vi "Housekeeping of Plugins.vi"(8 "error in (no error)":errorcluster, 11 "CIFPluginManager in":refnum<class "CIFPluginManager.lvclass">) -> (0 "error out":errorcluster)   [LabVIEW 2021, in "CIFPluginManager.lvclass"]
uses:
  CIFPluginManager.lvclass
  CIFPluginManager.lvclass/CIFPluginManager.ctl
  <vilib>/Utility/miscctls.llb/LVMapReplaceAction.ctl
  <vilib>/CIF Foundation/CIF Utilities/Time/System Time/LabVIEW Time to TAI Time.vi
  <vilib>/CIF Foundation/CIF Utilities/Time/Time_CIF_U.lvlib
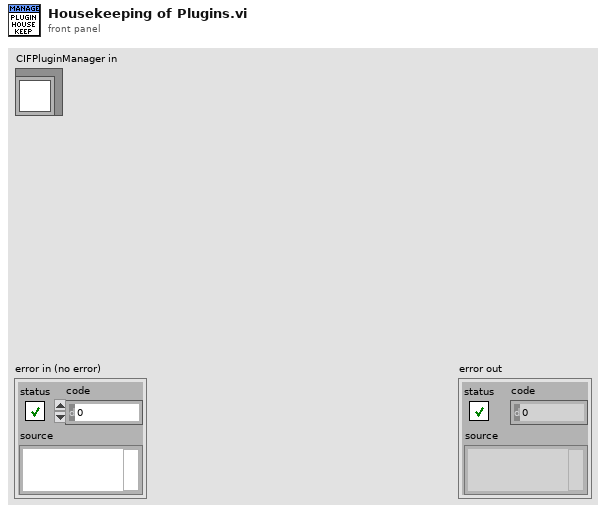
[diagram p1: front panel]
types:
  T1 = typedef "LVMapReplaceAction.ctl" = enum32{"Modify Entry only if found", "Add or Modify Entry", "Delete Entry"}
  T2 = typedef "CIFPluginManager.lvclass/Plugin Management Data Map.ctl" = map{string, T3}
  T3 = typedef "CIFPluginManager.lvclass/Plugin Management Data.ctl" = cluster{"vi reference":refnum<vi>, "gRPC ID":T4, "Plugin Type":string, "Unique Name":string, "gRPC Port":i32, "Version":T5, "Load Timestamp":i64, "Unload Timestamp":i64, "Unloading":bool, "Ready for removal":bool, "status":T6}
  T4 = typedef "grpc-lvsupport-release.lvlib/grpcId.ctl" = u64
  T5 = typedef "CIFCoreCommon.lvlib/Version.ctl" = cluster{"Major":i32, "Minor":i32, "Fix":i32, "Build":i32}
  T6 = typedef "CIF_Manager_server.lvlib/cif_plugincore_StatusData.ctl" = cluster{"state":T7, "timing_statistics":T8, "fifo_statistics":T10, "error":T11, "monitor_doubles":T12, "monitor_u64s":T13, "monitor_i64s":T14}
  T7 = typedef "CIF_Manager_server.lvlib/cif_plugincore_StatusData_State.ctl" = enum32{"NULL", "CREATING", "LISTENING", "RUNNING", "CLEANINGUP", "DESTROYING"}
  T8 = typedef "CIF_Manager_server.lvlib/cif_plugincore_TimingStatistics.ctl" = cluster{"period":T9, "wake_error":T9, "execute":T9, "housekeep":T9, "idle":T9, "cleanup":T9, "custom_1":T9, "custom_2":T9}
  T9 = typedef "CIF_Manager_server.lvlib/cif_common_TimingStats.ctl" = cluster{"max":i64, "min":i64, "avg":dbl}
  T10 = typedef "CIF_Manager_server.lvlib/cif_plugincore_FifoStatistics.ctl" = cluster{"from_t0":T9, "from_previous_plugin":T9, "output_error":T9}
  T11 = typedef "CIF_Manager_server.lvlib/cif_plugincore_Error.ctl" = cluster{"status":bool, "code":i32}
  T12 = typedef "CIF_Manager_server.lvlib/cif_plugincore_MonitorDoubles.ctl" = cluster{"double_1":dbl, "double_2":dbl, "double_3":dbl, "double_4":dbl}
  T13 = typedef "CIF_Manager_server.lvlib/cif_plugincore_MonitorU64.ctl" = cluster{"u64_1":u64, "u64_2":u64, "u64_3":u64, "u64_4":u64}
  T14 = typedef "CIF_Manager_server.lvlib/cif_plugincore_MonitorI64.ctl" = cluster{"i64_1":i64, "i64_2":i64, "i64_3":i64, "i64_4":i64}
  T15 = typedef "Plugin Management Data Map.ctl" = map{string, T3}
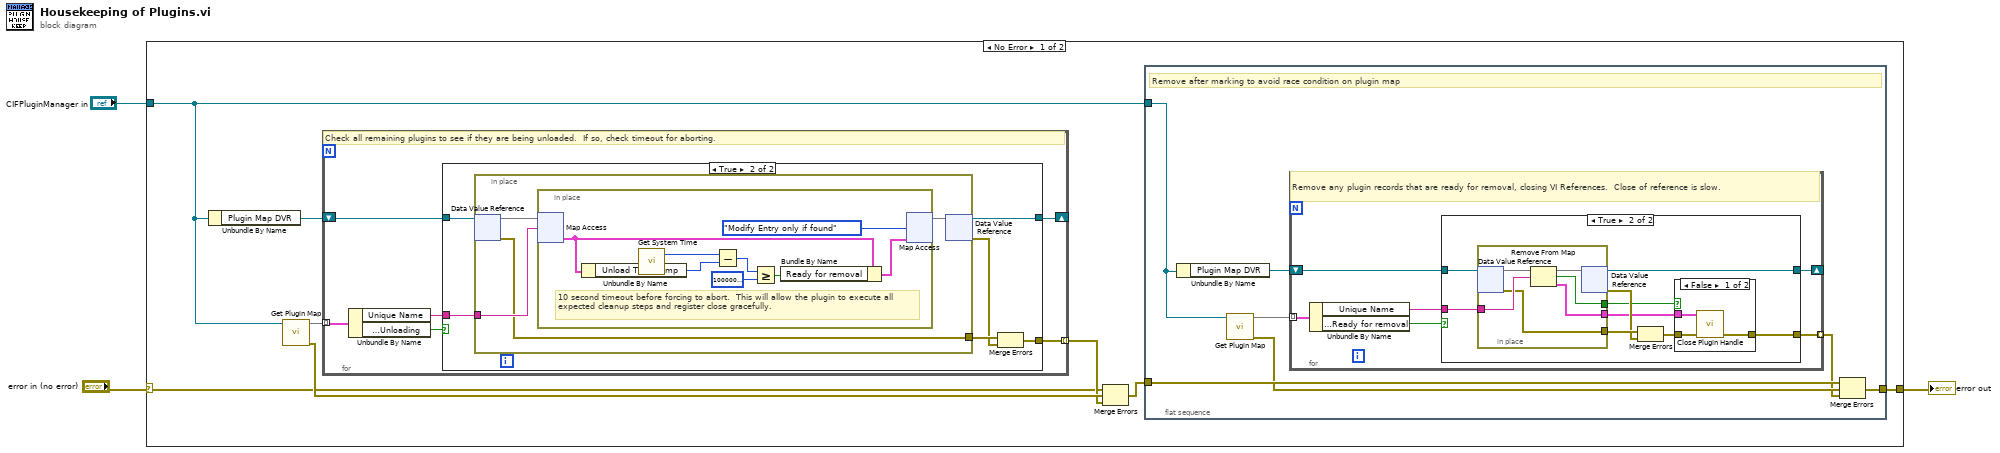
[diagram p0: block diagram]
diagram:
  n1 = case shown="No Error" "error in (no error)" {
    selector: "error in (no error)" -> [w6 w70]
    tunnel: [w4 w70] -> w2
    tunnel: "CIFPluginManager in" -> [w9 _]
    frame No Error {
      n2 = Unbundle By Name(w9) -> ("Plugin Map DVR"=w10:refnum<data-value>)
      n3 = call "Get Plugin Map.vi"("CIFPluginManager in"=w9) -> ("error out"=w8:errorcluster, "Plugin Map"=w11:T2)  [unwired: 9 in]
      n4 = for {
        tunnel: w11 -> [w50] mode=indexing
        shift-right: [w46] -> _
        shift-left: w10 -> [w49]
        tunnel: [w45] -> w7 mode=indexing
        # "Check all remaining plugins to see if they are being unloaded.  If so, check timeout for aborting."
        n5 = Unbundle By Name(w50) -> ("Unique Name"=w48:string, "Plugin Management Data.Unloading"=w47:bool)
        n6 = case shown="True" w47 {
          tunnel: w49 -> [w51 w56]
          tunnel: w48 -> [_ w57]
          tunnel: [w51 w53] -> w46
          tunnel: [_ w52] -> w45
          frame False {
          }
          frame True {
            n7 = in-place {
              in-place-border: w57 -> [w61]
              in-place-border: [w58] -> w55
              n8 = in-place-dvr #1(w56) -> (w60:T15, w58:errorcluster)
              n9 = in-place {
                # "10 second timeout before forcing to abort.  This will allow the plugin to execute all expected cleanup steps and register close gracefully."
                n10 = in-place-map #2(w60, w61) -> (w67:T3)  [unwired: 1 in, 1 out]
                n11 = Unbundle By Name(w67) -> ("Unload Timestamp"=w68:i64)
                n12 = call <vilib>:"Get System Time.vi"() -> ("Time (ns)"=w62:i64)  [unwired: 5 in]
                n13 = Subtract(x=w62, y=w68) -> (x-y=w66:i64)
                n14 = Greater Or Equal?(x=w66, y=i64 10000000000) -> (x >= y?=w64:bool)
                n15 = Bundle By Name(cluster=w67, "Ready for removal"=w64) -> (w63:T3)
                n16 = in-place-map #2(w63, LVMapReplaceAction."Modify Entry only if found" ("action")) -> (w59:T15)  [unwired: 2 out]
              }
              n17 = in-place-dvr #1(w59) -> (w53:refnum<data-value>, w54:errorcluster)
            }
            n18 = Merge Errors(w55, w54) -> (w52:errorcluster)
          }
        }
      }
      n19 = Merge Errors(w6, w8, w7) -> (w5:errorcluster)
      n20 = flat-sequence {
        tunnel: [w12] -> w4
        tunnel: w9 -> [w17]
        tunnel: w5 -> [w16]
        frame #0 {
          # "Remove after marking to avoid race condition on plugin map"
          n21 = Unbundle By Name(w17) -> ("Plugin Map DVR"=w18:refnum<data-value>)
          n22 = call "Get Plugin Map.vi"("CIFPluginManager in"=w17) -> ("error out"=w14:errorcluster, "Plugin Map"=w15:T2)  [unwired: 9 in]
          n23 = for {
            tunnel: w15 -> [w24] mode=indexing
            shift-right: [w20] -> _
            shift-left: w18 -> [w23]
            tunnel: [w19] -> w13 mode=indexing
            # "Remove any plugin records that are ready for removal, closing VI References.  Close of reference is slow."
            n24 = Unbundle By Name(w24) -> ("Unique Name"=w22:string, "Plugin Management Data.Ready for removal"=w21:bool)
            n25 = case shown="True" w21 {
              tunnel: w23 -> [w25 w33]
              tunnel: w22 -> [_ w34]
              tunnel: [w25 w32] -> w20
              tunnel: [_ w28] -> w19
              frame False {
              }
              frame True {
                n26 = in-place {
                  in-place-border: w34 -> [w44]
                  in-place-border: [w42] -> w31
                  in-place-border: [w40] -> w27
                  in-place-border: [w39] -> w26
                  n27 = in-place-dvr #3(w33) -> (w43:T15, w42:errorcluster)
                  n28 = Remove From Map(10:w44, 11:w43) -> (1:w40:T3, 2:w39:bool, 3:w41:T15)
                  n29 = in-place-dvr #3(w41) -> (w32:refnum<data-value>, w30:errorcluster)
                }
                n30 = Merge Errors(w31, w30) -> (w29:errorcluster)
                n31 = case shown="False" w26 {
                  tunnel: w29 -> [w37 w38]
                  tunnel: [w36 w38] -> w28
                  tunnel: w27 -> [w35 _]
                  frame False {
                    n32 = call "Close Plugin Handle.vi"("error in (no error)"=w37, "Plugin Management Data"=w35) -> ("error out"=w36:errorcluster)  [unwired: 9 in]
                  }
                  frame True {
                  }
                }
              }
            }
          }
          n33 = Merge Errors(w16, w14, w13) -> (w12:errorcluster)
        }
      }
    }
    frame Error {
    }
  }
  "error out" <- w2
